vi "processContactData_MFP3D_Lucy.vi"(0 "tdms file":refnum<k34>, 1 "data":dbl[](array[numeric]), 2 "tip voltage":dbl, 3 "lvdt":cluster{dbl, dbl, dbl, dbl, dbl, dbl}, 4 "time stamp":timestamp) -> (5 "z":dbl, 6 "tdms file out":refnum<k34>, 7 "x":dbl, 8 "y":dbl, 9 "deflection":dbl format="%#_13g", 10 "tip voltage":dbl)   [LabVIEW 2020]
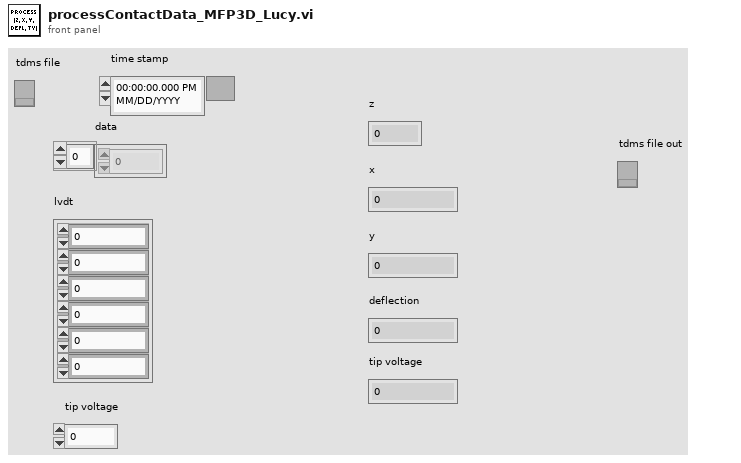
[diagram p1: front panel]
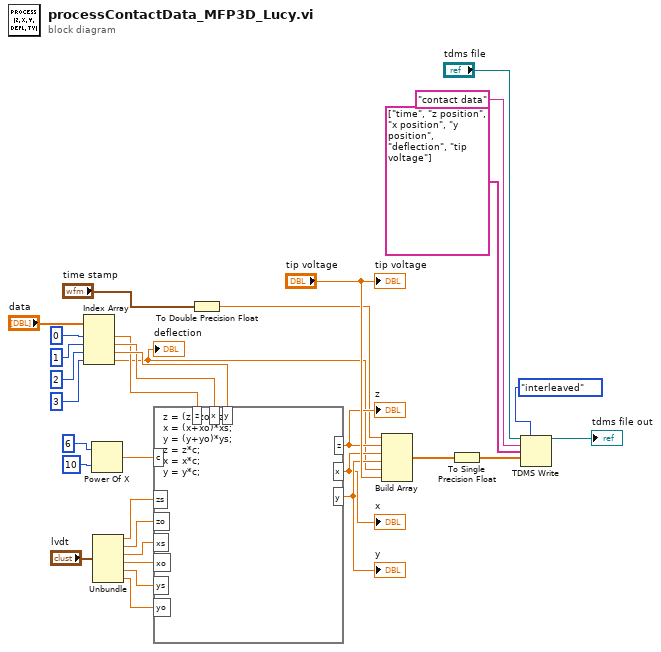
[diagram p0: block diagram]
diagram:
  n1 = Index Array(array="data", index #1=0, index #2=1, index #3=2, index #4=3) -> (element #1=w15:dbl, element #2=w16:dbl, element #3=w17:dbl, element #4=w9:dbl)
  "deflection" <- w9
  n2 = Power Of X(1:10, 2:6) -> (0:w28:dbl)
  n3 = Unbundle("lvdt") -> (w20:dbl, w21:dbl, w22:dbl, w23:dbl, w24:dbl, w25:dbl)
  n4 = formula code="z = (z+zo)*zs;\nx = (x+xo)*xs;\ny = (y+yo)*ys;\nz = z*c;\nx = x*c;\ny = y*c;"("z"=w15, "x"=w16, "y"=w17, "zo"=w21, "xs"=w22, "xo"=w23, "ys"=w24, "zs"=w20, "yo"=w25, "c"=w28) -> ("z"=w29:dbl, "x"=w30:dbl, "y"=w31:dbl)
  "y" <- w31
  "x" <- w30
  "z" <- w29
  n5 = To Double Precision Float(number="time stamp") -> (double precision float=w18:dbl)
  n6 = Build Array(w18, w29, w30, w31, w9, "tip voltage") -> (w4:dbl[])
  n7 = To Single Precision Float(number=w4) -> (single precision float=w3:sgl[])
  n8 = TDMS Write(0:"tdms file", 1:enum16{"decimated", "interleaved"}."interleaved" ("data layout (0:decimated)"), 5:"contact data", 7:string[] ["time", "z position", "x position", "y position", "deflection", "tip voltage"], 9:w3) -> (4:→"tdms file out":refnum<k34>)  [unwired: 1 in, 3 out]
  "tip voltage" <- "tip voltage"
